vi "Tabulate 2D Array.vi"(10 "Tabulation Column":i32, 11 "Input Array":string[][](array[string])) -> (3 "Tabulation":string[][](array[string]))   [LabVIEW 2010]
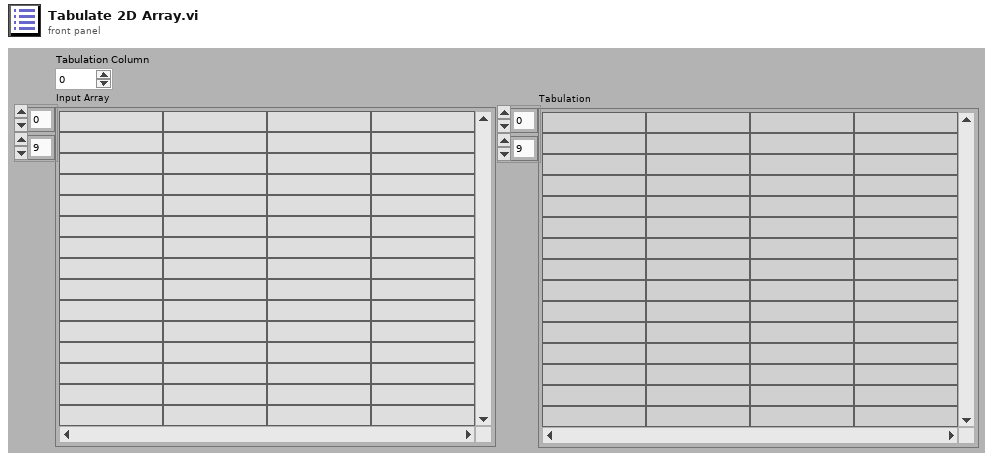
[diagram p1: front panel]
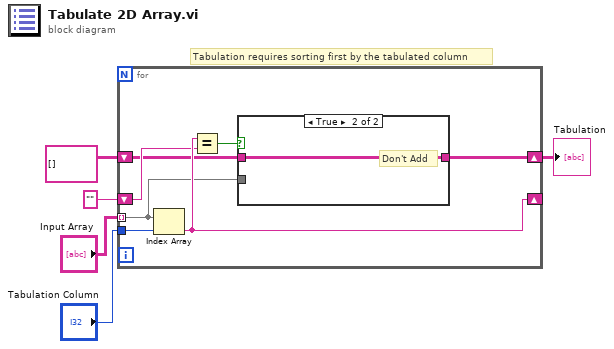
[diagram p0: block diagram]
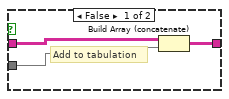
[diagram p2: hidden frame]
diagram:
  # "Tabulation requires sorting first by the tabulated column"
  n1 = for {
    shift-right: [w11] -> _
    shift-left: "" ("String") -> [w10]
    tunnel: "Input Array" -> [w8] mode=indexing
    tunnel: "Tabulation Column" -> [w12]
    shift-right: [w7] -> w1
    shift-left: string[][] [] -> [w6]
    n2 = Index Array(array=w8, index=w12) -> (element=w11:string)
    n3 = Equal?(x=w11, y=w10) -> (x = y?=w9:bool)
    n4 = case shown="True" w9 {
      tunnel: w8 -> [w15 _]
      tunnel: [w14 w16] -> w7
      tunnel: w6 -> [w13 w16]
      frame False {
        # "Add to tabulation"
        n5 = Build Array (concatenate)(w13, w15) -> (w14:string[][])
      }
      frame True {
        # "Don't Add"
      }
    }
  }
  "Tabulation" <- w1
